vi "Autonomous Independent.vi"() -> ()   [LabVIEW 2016]
doc: "This VI is called when autonomous begins, and will automatically be terminated when autonomous ends. You can carry out timed or sensor driven robot movement independently without needing to return to the caller."
uses:
  <vilib>/Rock Robotics/WPI/Solenoid/WPI_SolenoidValue.ctl
  <vilib>/Rock Robotics/Network Tables/NT Read String.vi
  Robot Global Data.vi
  <vilib>/Rock Robotics/WPI/Solenoid/WPI_SolenoidSetEnum.vi
  <vilib>/Rock Robotics/WPI/Utilities/WPI_GetSetVariantRefNum.vi
  <vilib>/addons/control/pid/pid.llb/PID (DBL).vi
  <vilib>/addons/control/pid/NI_PID_pid.lvlib
  navX Library v2/navX Library v2.lvlib
panel:
  in  "ForwardPID":T1={"proportional gain (Kc)"=0.001, "integral time (Ti, min)"=0.1, "derivative time (Td, min)"=0.0}
  out "DriveStraight":T2(graph)
  in  "Center":dbl=180.0 format="%#_13g"
  in  "MOE":dbl=25.0 format="%#_13g"
  in  "Speed 2":dbl=0.45 format="%#_13g"
  in  "PID gains L":T1={"proportional gain (Kc)"=1.5e-05, "integral time (Ti, min)"=1e-07, "derivative time (Td, min)"=0.0} {"derivative time (Td, min)" format="%.3f"; "integral time (Ti, min)" format="%.6f"; "proportional gain (Kc)" format="%.6f"}
  in  "PID gains R":T1={"proportional gain (Kc)"=1.5e-05, "integral time (Ti, min)"=1e-07, "derivative time (Td, min)"=0.0} {"derivative time (Td, min)" format="%.3f"; "integral time (Ti, min)" format="%.6f"; "proportional gain (Kc)" format="%.6f"}
  in  "Range":cluster{"output high":dbl, "output low":dbl}={"output high"=1.0, "output low"=-1.0} {"output low" format="%.2f"; "output high" format="%.2f"}
  out "Right V":cluster{"output":dbl, dbl, "Numeric":dbl}(graph)
  out "Left V":cluster{"output":dbl, dbl, "Numeric":dbl}(graph)
  in  "Speed":dbl=1.0 format="%#_13g"
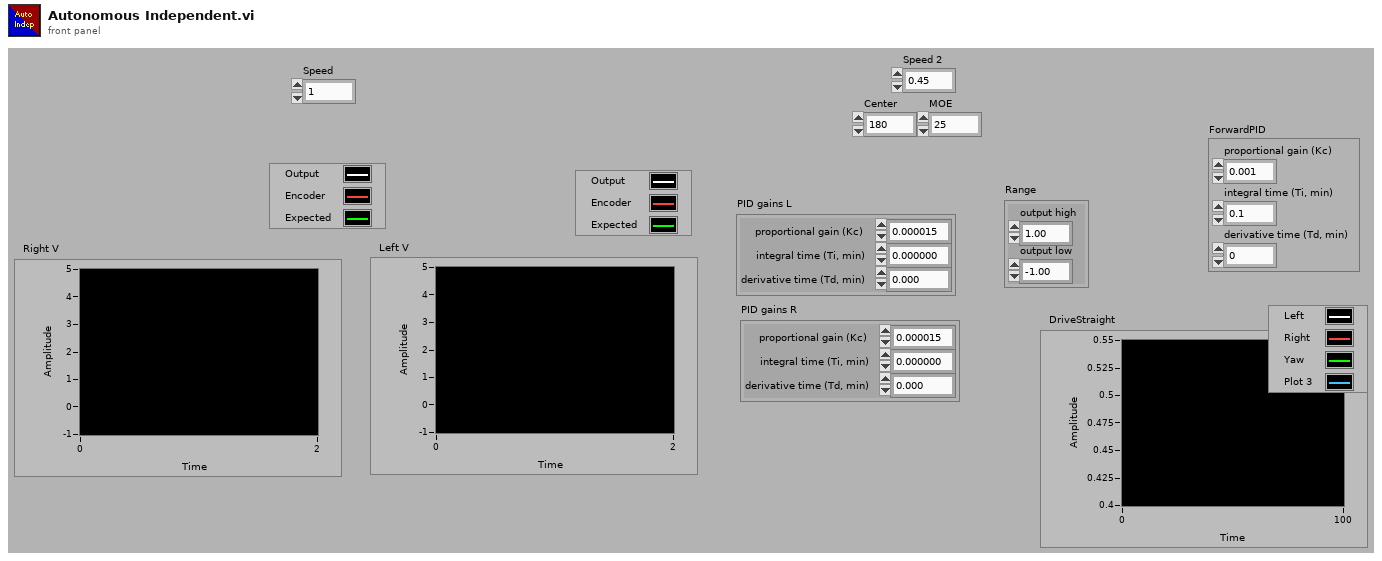
[diagram p1: front panel]
types:
  T1 = cluster{"proportional gain (Kc)":dbl, "integral time (Ti, min)":dbl, "derivative time (Td, min)":dbl}
  T2 = cluster{"[0]":dbl, "[1]":dbl, "[2]":dbl, "[3]":dbl, "[4]":dbl, "[5]":dbl, "[6]":dbl, "[7]":dbl, "[8]":dbl}
  T3 = typedef "WPI_SolenoidValue.ctl" = enum16{"Off", "On", "Forward", "Reverse"}
  T4 = typedef "WPI_SolenoidDevRef.ctl" = cluster{"DevStatus":errorcluster, "Pneumatics Control Module":u8, "Forward Solenoid Channel":T5, "Reverse Solenoid Channel":T5}
  T5 = typedef "WPI_SolenoidChannel.ctl" = enum8{"Solenoid 0", "Solenoid 1", "Solenoid 2", "Solenoid 3", "Solenoid 4", "Solenoid 5", "Solenoid 6", "Solenoid 7", "Invalid"}
  T6 = typedef "WPI_RobotDriveDevRef.ctl" = cluster{"DevStatus":errorcluster, "Motors[]":T7[], "Square Inputs":bool, "Max Output":dbl}
  T7 = typedef "WPI_MotorControlDeviceRef.ctl" = cluster{"DeviceStatus":errorcluster, "Type":T8, "PWM":cluster{"PWM Channel":T9, "DeadBand":T10}, "CAN":cluster{"Device Number":u8, "SetOutput VI Ref":variant, "GetOutput VI Ref":variant, "Enable VI Ref":variant, "Disable VI Ref":variant, "Data":variant}, "Invert":bool}
  T8 = typedef "WPI_MotorControlType.ctl" = enum16{"PWM", "CAN"}
  T9 = typedef "FPGA_DIOPWMChannel.ctl" = enum8{"PWM 0", "PWM 1", "PWM 2", "PWM 3", "PWM 4", "PWM 5", "PWM 6", "PWM 7", "PWM 8", "PWM 9", "PWM MXP 0", "PWM MXP 1", "PWM MXP 2", "PWM MXP 3", "PWM MXP 4", "PWM MXP 5", "PWM MXP 6", "PWM MXP 7", "PWM MXP 8", "PWM MXP 9", "Invalid"}
  T10 = typedef "WPI_PWMDeadband.ctl" = cluster{"Name":string, "maxPositivePwm":i32, "minPositivePwm":i32, "centerPwm":i32, "maxNegativePwm":i32, "minNegativePwm":i32, "angularRange":u16}
  T11 = typedef "navX Library v2.lvlib/Z900_navX_DeviceTypeDef.ctl" = cluster{"Interface":cluster{"Protocol":T12, "Update Rate (4Hz-100Hz)":u8, "navX Open TypeDef":variant}, "Notify Packet":refnum<notifier>, "Loop VI Refnum":refnum<vi>, "Ready to Close Occurrence Refnum":refnum<k4>}
  T12 = typedef "navX Library v2.lvlib/Z900_navX_ProtocolTypeDef.ctl" = enum16{"SERIAL", "I2C", "SPI"}
  T13 = typedef "WPI_EncoderDevRef.ctl" = cluster{"DevStatus":errorcluster, "EncoderIndex":T14, "CounterIndex":T15, "DistancePerCount":dbl, "Decoding Type":T16}
  T14 = typedef "FPGA_EncoderIdx.ctl" = enum8{"Enc 0", "Enc 1", "Enc 2", "Enc 3", "Enc 4", "Enc 5", "Enc 6", "Enc 7", "Invalid"}
  T15 = typedef "FPGA_CounterCtrSystemIndex.ctl" = enum8{"Ctr 0", "Ctr 1", "Ctr 2", "Ctr 3", "Ctr 4", "Ctr 5", "Ctr 6", "Ctr 7", "Invalid"}
  T16 = typedef "WPI_EncoderType.ctl" = enum16{"1x", "2x", "4x"}
  T17 = cluster{"Yaw":dbl, "Roll":dbl, "Pitch":dbl, "Heading":dbl, "Fused Heading":dbl}
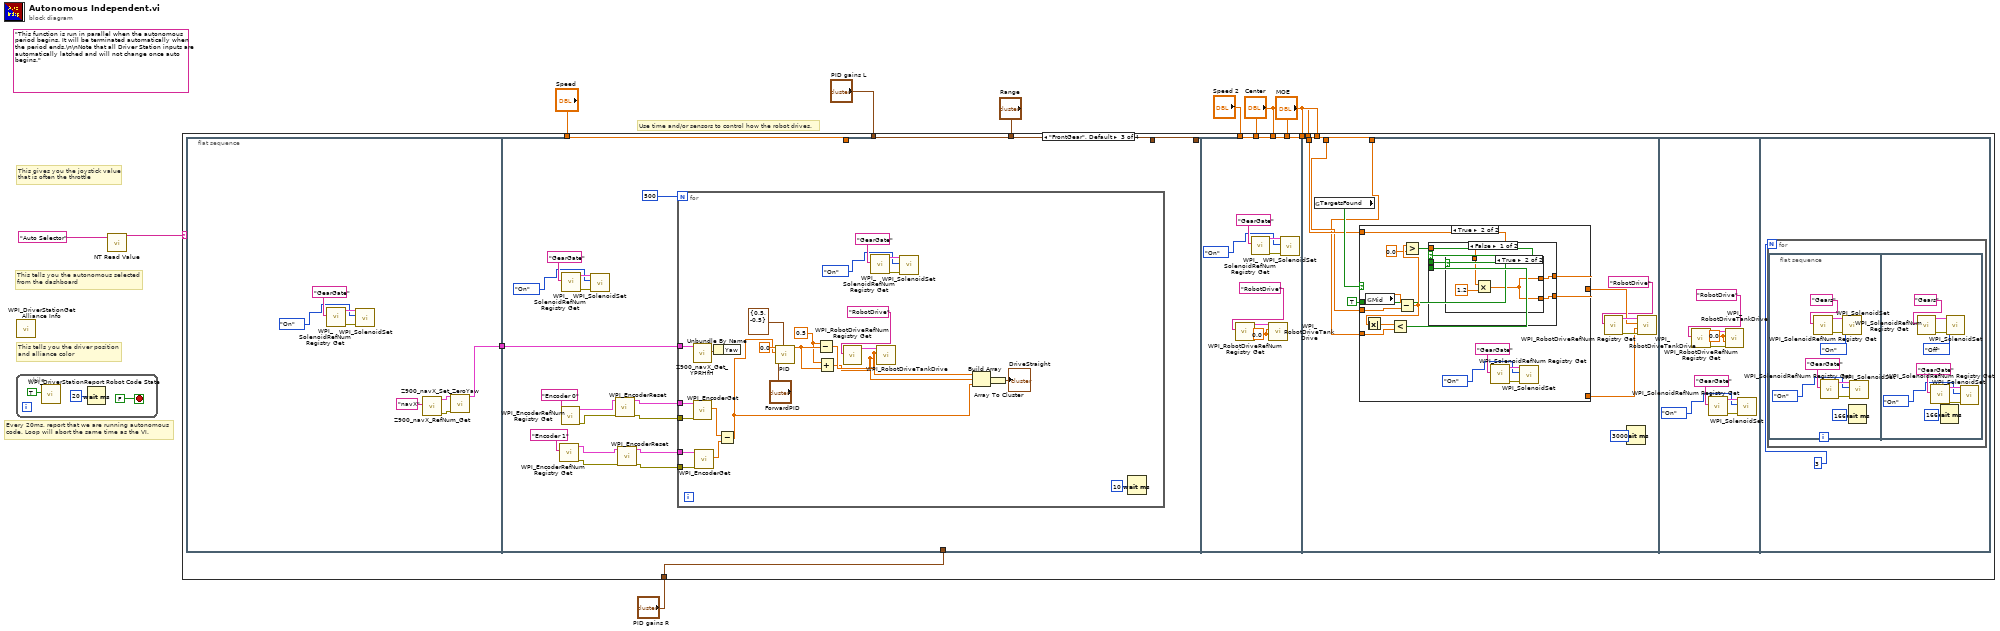
[diagram p0: block diagram]
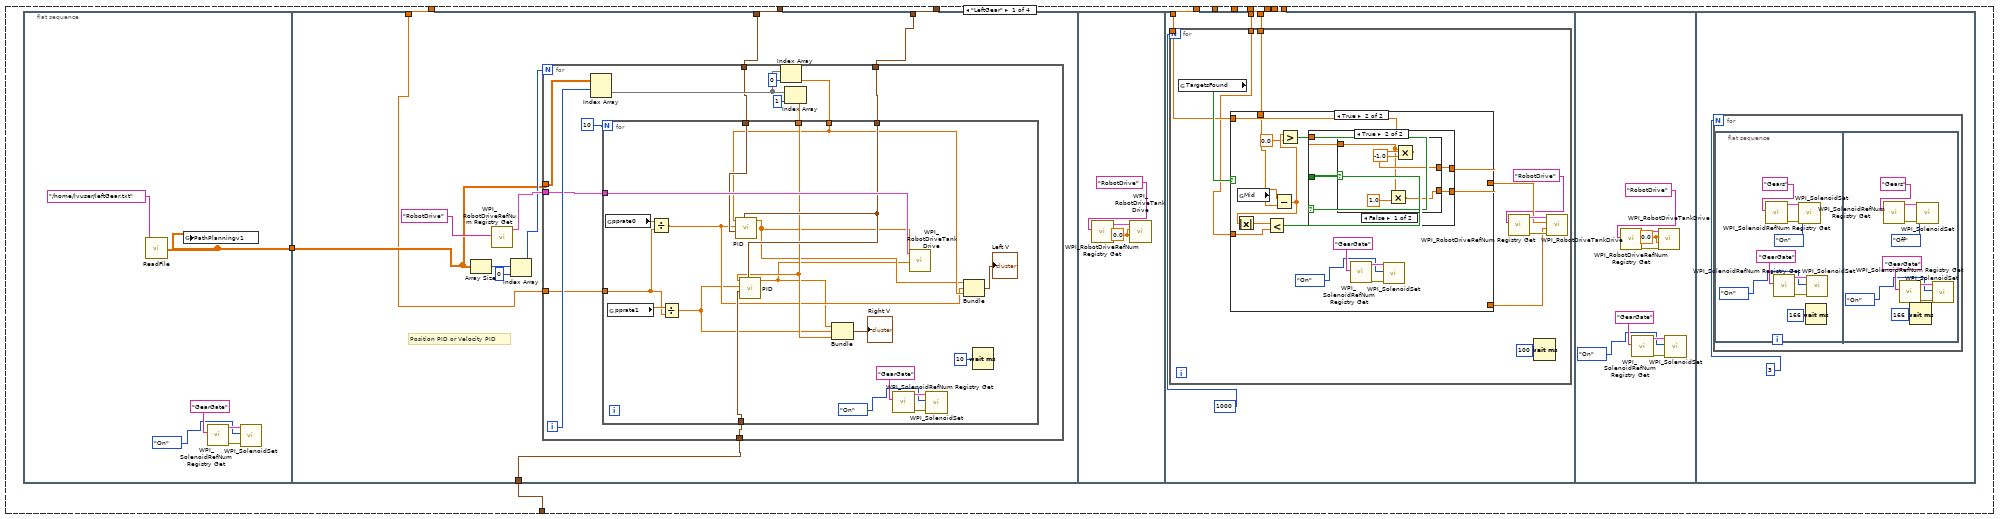
[diagram p2: hidden frame]
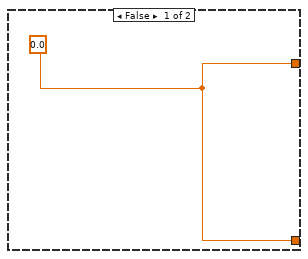
[diagram p3: hidden frame]
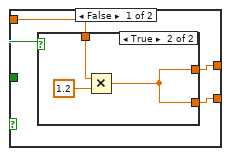
[diagram p4: hidden frame]
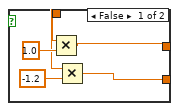
[diagram p5: hidden frame]
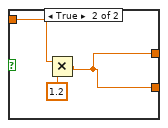
[diagram p6: hidden frame]
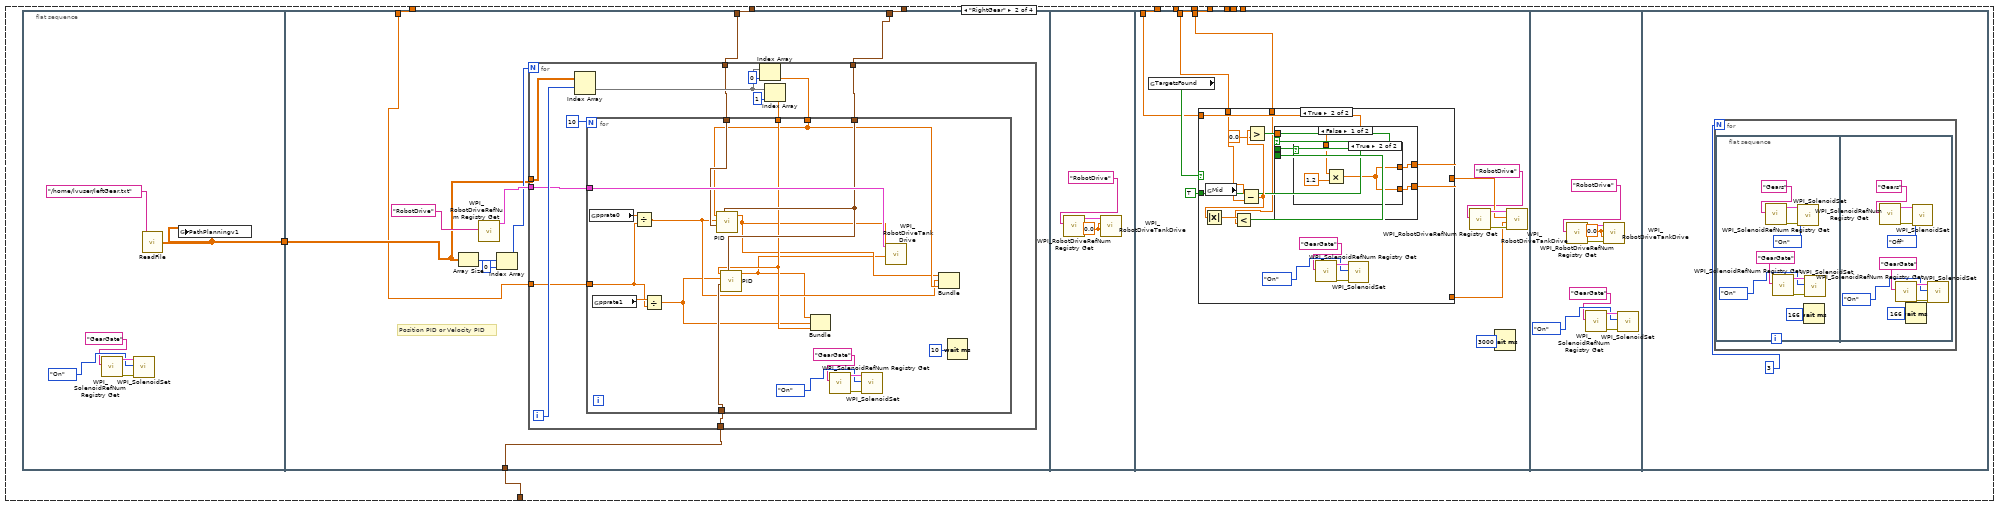
[diagram p7: hidden frame]
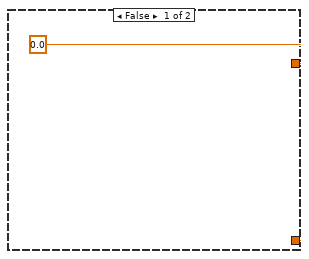
[diagram p8: hidden frame]
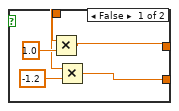
[diagram p9: hidden frame]
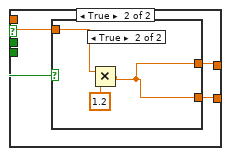
[diagram p10: hidden frame]
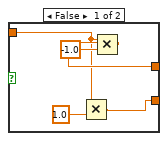
[diagram p11: hidden frame]
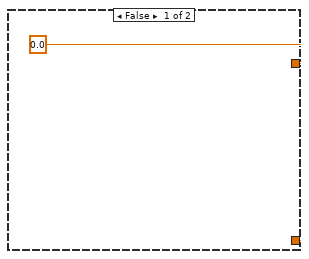
[diagram p12: hidden frame]
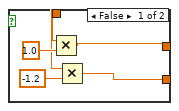
[diagram p13: hidden frame]
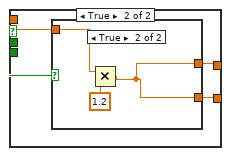
[diagram p14: hidden frame]
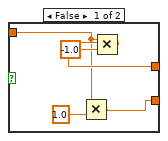
[diagram p15: hidden frame]
diagram:
  (unwired) "This function is run in parallel when the autonomous period begins. It will be terminated automatically when the period ends.\n\nNote that all Driver Station inputs are automatically latched and will not change once auto begins."
  # "This tells you the autonomous selected\nfrom the dashboard"
  # "Every 20ms, report that we are running autonomous\ncode. Loop will abort the same time as the VI."
  # "This gives you the joystick value\nthat is often the throttle"
  # "Use time and/or sensors to control how the robot drives."
  # "This tells you the driver position\nand alliance color"
  n1 = while {
    stop <- FALSE stop-if-true
    n2 = call <vilib>:"WPI_DriverStationReport Robot Code State.vi"("Autonomous"=TRUE) -> ()  [unwired: 10 in, 1 out]
    n3 = Wait (ms)(milliseconds to wait=u32 20) -> ()  [unwired: 1 out]
  }
  n4 = call <vilib>:"WPI_DriverStationGet Alliance Info.vi"() -> ()  [unwired: 12 out]
  n5 = call-poly <vilib>:"NT Read Value.vi"("Name"="Auto Selector") -> ("String"=w8:string)  [unwired: 9 in, 1 out]
  n6 = case shown="\"FrontGear\", Default" w8 {
    tunnel: "Range" -> [w19 w160 w298 _]
    tunnel: "PID gains L" -> [w18 w159 w297 _]
    tunnel: "Speed 2" -> [w17 w157 w296 _]
    tunnel: "Center" -> [w16 _ _ _]
    tunnel: "MOE" -> [w15 _ _ _]
    tunnel: "Speed" -> [w14 w158 w293 _]
    tunnel: "Center" -> [_ w156 _ _]
    tunnel: "MOE" -> [_ w155 _ _]
    tunnel: "Center" -> [_ _ w295 _]
    tunnel: "MOE" -> [_ _ w294 _]
    tunnel: "PID gains R" -> [w13 w154 w292 _]
    frame "LeftGear" {
      n7 = flat-sequence {
        tunnel: [w25] -> w20
        tunnel: w20 -> [w31]
        tunnel: w19 -> [w30]
        tunnel: w18 -> [w29]
        tunnel: w14 -> [w28]
        tunnel: w13 -> [w27]
        tunnel: w17 -> [w76]
        tunnel: w16 -> [w75]
        tunnel: w15 -> [w74]
        frame #0 {
          n8 = call "ReadFile.vi"("Name"="/home/lvuser/leftGear.txt") -> ("Array - Numeric"=w25:dbl[][])
          n9 = global write "Robot Global Data.vi" "PathPlanningv1"(w25) -> ()
          n10 = call <vilib>:"WPI_SolenoidRefNum Registry Get.vi"("refnum name"="GearGate") -> ("error out"=w24:errorcluster, "SolenoidDevRef"=w23:T4)  [unwired: 9 in]
          n11 = call-poly <vilib>:"WPI_SolenoidSet.vi"("error in (no error)"=w24, "Value"=WPI_SolenoidValue."On", "SolenoidDevRef"=w23) -> ()  [unwired: 7 in, 2 out]
        }
        frame #1 {
          # "Position PID or Velocity PID"
          n12 = Array Size(array=w31) -> (size(s)=w36:i32[])
          n13 = call <vilib>:"WPI_RobotDriveRefNum Registry Get.vi"("refnum name"="RobotDrive") -> ("RobotDriveDevRef"=w33:T6)  [unwired: 9 in, 1 out]
          n14 = Index Array(array=w36, index=0) -> (element=w32:i32)
          n15 = for {
            N: w32 -> [_]
            tunnel: w31 -> [w46]
            tunnel: w27 -> [w41]
            tunnel: w29 -> [w40]
            tunnel: w30 -> [w39]
            tunnel: w33 -> [w38]
            tunnel: w28 -> [w37]
            i -> [w43]
            n16 = Index Array(array=w46, index (row)=w43) -> (element=w49:dbl[])  [unwired: 1 in]
            n17 = Index Array(array=w49, index=0) -> (element=w45:dbl)
            n18 = Index Array(array=w49, index=1) -> (element=w44:dbl)
            n19 = for {
              N: 10 -> [_]
              tunnel: w45 -> [w63]
              tunnel: w44 -> [w64]
              tunnel: w41 -> [w67]
              tunnel: w40 -> [w66]
              tunnel: w39 -> [w65]
              tunnel: w38 -> [w68]
              tunnel: w37 -> [w56]
              n20 = global read "Robot Global Data.vi" "pprate0"() -> (w60:dbl)
              n21 = global read "Robot Global Data.vi" "pprate1"() -> (w57:dbl)
              n22 = Divide(x=w60, y=w56) -> (x/y=w59:dbl)
              n23 = Divide(x=w57, y=w56) -> (x/y=w58:dbl)
              n24 = call-poly <vilib>:"PID.vi"("output range"=w65, "PID gains"=w66, "process variable"=w59, "setpoint"=w63) -> ("output"=w55:dbl)  [unwired: 6 in, 1 out]
              n25 = call-poly <vilib>:"PID.vi"("output range"=w65, "PID gains"=w67, "process variable"=w58, "setpoint"=w64) -> ("output"=w54:dbl)  [unwired: 6 in, 1 out]
              n26 = Bundle("output"=w54, w58, "Numeric"=w64) -> (→"Right V":cluster{"output":dbl, dbl, "Numeric":dbl})  [unwired: 1 in]
              n27 = call <vilib>:"WPI_SolenoidRefNum Registry Get.vi"("refnum name"="GearGate") -> ("error out"=w53:errorcluster, "SolenoidDevRef"=w52:T4)  [unwired: 9 in]
              n28 = call <vilib>:"WPI_RobotDriveTankDrive.vi"("Right axis value"=w54, "Left axis value"=w55, "RobotDriveDevRef"=w68) -> ()  [unwired: 6 in, 3 out]
              n29 = call-poly <vilib>:"WPI_SolenoidSet.vi"("error in (no error)"=w53, "Value"=WPI_SolenoidValue."On", "SolenoidDevRef"=w52) -> ()  [unwired: 7 in, 2 out]
              n30 = Bundle("output"=w55, w59, "Numeric"=w63) -> (→"Left V":cluster{"output":dbl, dbl, "Numeric":dbl})  [unwired: 1 in]
              n31 = Wait (ms)(milliseconds to wait=10) -> ()  [unwired: 1 out]
            }
          }
        }
        frame #2 {
          w71 = 0.0 ("Right axis value")
          n32 = call <vilib>:"WPI_RobotDriveRefNum Registry Get.vi"("refnum name"="RobotDrive") -> ("RobotDriveDevRef"=w72:T6)  [unwired: 9 in, 1 out]
          n33 = call <vilib>:"WPI_RobotDriveTankDrive.vi"("Right axis value"=w71, "Left axis value"=w71, "RobotDriveDevRef"=w72) -> ()  [unwired: 6 in, 3 out]
        }
        frame #3 {
          n34 = for {
            N: 1000 -> [_]
            tunnel: w76 -> [w79]
            tunnel: w75 -> [w78]
            tunnel: w74 -> [w77]
            n35 = global read "Robot Global Data.vi" "TargetsFound"() -> (w80:bool)
            n36 = case shown="True" w80 {
              tunnel: [w87 w99] -> w83
              tunnel: [w87 w98] -> w84
              tunnel: w79 -> [_ w94]
              tunnel: w78 -> [_ w93]
              tunnel: w77 -> [_ w92]
              frame False {
                w87 = 0.0
              }
              frame True {
                n37 = global read "Robot Global Data.vi" "Mid"() -> (w102:dbl)
                n38 = Subtract(x=w102, y=w93) -> (x-y=w96:dbl)
                n39 = Absolute Value(x=w96) -> (abs(x)=w101:dbl)
                n40 = Less?(x=w101, y=w92) -> (x < y?=w100:bool)
                n41 = Greater?(x=w96, y=0.0) -> (0:w97:bool)
                n42 = case shown="True" w97 {
                  tunnel: w100 -> [w103 w118]
                  tunnel: [w104 w116] -> w99
                  tunnel: [w105 w117] -> w98
                  tunnel: w94 -> [w106 w115]
                  frame False {
                    n43 = case shown="True" w103 {
                      tunnel: [w111 w114] -> w105
                      tunnel: [w109 w114] -> w104
                      tunnel: w106 -> [w107 w112]
                      frame False {
                        n44 = Multiply(x=w107, y=1.0) -> (x*y=w111:dbl)
                        n45 = Multiply(x=w107, y=-1.2) -> (x*y=w109:dbl)
                      }
                      frame True {
                        n46 = Multiply(x=w112, y=1.2) -> (x*y=w114:dbl)
                      }
                    }
                  }
                  frame True {
                    n47 = case shown="False" w118 {
                      tunnel: [w123 w126] -> w117
                      tunnel: [w121 w126] -> w116
                      tunnel: w115 -> [w119 w124]
                      frame False {
                        n48 = Multiply(x=w119, y=1.0) -> (x*y=w121:dbl)
                        n49 = Multiply(x=w119, y=-1.0) -> (x*y=w123:dbl)
                      }
                      frame True {
                        n50 = Multiply(x=w124, y=1.2) -> (x*y=w126:dbl)
                      }
                    }
                  }
                }
                n51 = call <vilib>:"WPI_SolenoidRefNum Registry Get.vi"("refnum name"="GearGate") -> ("error out"=w91:errorcluster, "SolenoidDevRef"=w90:T4)  [unwired: 9 in]
                n52 = call-poly <vilib>:"WPI_SolenoidSet.vi"("error in (no error)"=w91, "Value"=WPI_SolenoidValue."On", "SolenoidDevRef"=w90) -> ()  [unwired: 7 in, 2 out]
              }
            }
            n53 = call <vilib>:"WPI_RobotDriveRefNum Registry Get.vi"("refnum name"="RobotDrive") -> ("error out"=w85:errorcluster, "RobotDriveDevRef"=w86:T6)  [unwired: 9 in]
            n54 = Wait (ms)(milliseconds to wait=100) -> ()  [unwired: 1 out]
            n55 = call <vilib>:"WPI_RobotDriveTankDrive.vi"("error in (no error)"=w85, "Right axis value"=w83, "Left axis value"=w84, "RobotDriveDevRef"=w86) -> ()  [unwired: 5 in, 3 out]
          }
        }
        frame #4 {
          w132 = 0.0 ("Left axis value")
          n56 = call <vilib>:"WPI_RobotDriveRefNum Registry Get.vi"("refnum name"="RobotDrive") -> ("error out"=w133:errorcluster, "RobotDriveDevRef"=w134:T6)  [unwired: 9 in]
          n57 = call <vilib>:"WPI_SolenoidRefNum Registry Get.vi"("refnum name"="GearGate") -> ("error out"=w130:errorcluster, "SolenoidDevRef"=w129:T4)  [unwired: 9 in]
          n58 = call <vilib>:"WPI_RobotDriveTankDrive.vi"("error in (no error)"=w133, "Right axis value"=w132, "Left axis value"=w132, "RobotDriveDevRef"=w134) -> ()  [unwired: 5 in, 3 out]
          n59 = call-poly <vilib>:"WPI_SolenoidSet.vi"("error in (no error)"=w130, "Value"=WPI_SolenoidValue."On", "SolenoidDevRef"=w129) -> ()  [unwired: 7 in, 2 out]
        }
        frame #5 {
          n60 = for {
            N: 3 -> [_]
            n61 = flat-sequence {
              frame #0 {
                n62 = call <vilib>:"WPI_SolenoidRefNum Registry Get.vi"("refnum name"="Gears") -> ("error out"=w144:errorcluster, "SolenoidDevRef"=w143:T4)  [unwired: 9 in]
                n63 = call <vilib>:"WPI_SolenoidRefNum Registry Get.vi"("refnum name"="GearGate") -> ("error out"=w139:errorcluster, "SolenoidDevRef"=w138:T4)  [unwired: 9 in]
                n64 = call-poly <vilib>:"WPI_SolenoidSet.vi"("error in (no error)"=w144, "Value"=WPI_SolenoidValue."On", "SolenoidDevRef"=w143) -> ()  [unwired: 7 in, 2 out]
                n65 = Wait (ms)(milliseconds to wait=166) -> ()  [unwired: 1 out]
                n66 = call-poly <vilib>:"WPI_SolenoidSet.vi"("error in (no error)"=w139, "Value"=WPI_SolenoidValue."On", "SolenoidDevRef"=w138) -> ()  [unwired: 7 in, 2 out]
              }
              frame #1 {
                n67 = call <vilib>:"WPI_SolenoidRefNum Registry Get.vi"("refnum name"="Gears") -> ("error out"=w153:errorcluster, "SolenoidDevRef"=w152:T4)  [unwired: 9 in]
                n68 = call <vilib>:"WPI_SolenoidRefNum Registry Get.vi"("refnum name"="GearGate") -> ("error out"=w148:errorcluster, "SolenoidDevRef"=w147:T4)  [unwired: 9 in]
                n69 = Wait (ms)(milliseconds to wait=166) -> ()  [unwired: 1 out]
                n70 = call-poly <vilib>:"WPI_SolenoidSet.vi"("error in (no error)"=w153, "Value"=WPI_SolenoidValue."Off", "SolenoidDevRef"=w152) -> ()  [unwired: 7 in, 2 out]
                n71 = call-poly <vilib>:"WPI_SolenoidSet.vi"("error in (no error)"=w148, "Value"=WPI_SolenoidValue."On", "SolenoidDevRef"=w147) -> ()  [unwired: 7 in, 2 out]
              }
            }
          }
        }
      }
    }
    frame "RightGear" {
      n72 = flat-sequence {
        tunnel: [w166] -> w161
        tunnel: w161 -> [w172]
        tunnel: w160 -> [w171]
        tunnel: w159 -> [w170]
        tunnel: w158 -> [w169]
        tunnel: w154 -> [w168]
        tunnel: w157 -> [w214]
        tunnel: w156 -> [w213]
        tunnel: w155 -> [w212]
        frame #0 {
          n73 = call <vilib>:"WPI_SolenoidRefNum Registry Get.vi"("refnum name"="GearGate") -> ("error out"=w165:errorcluster, "SolenoidDevRef"=w164:T4)  [unwired: 9 in]
          n74 = call-poly <vilib>:"WPI_SolenoidSet.vi"("error in (no error)"=w165, "Value"=WPI_SolenoidValue."On", "SolenoidDevRef"=w164) -> ()  [unwired: 7 in, 2 out]
          n75 = call "ReadFile.vi"("Name"="/home/lvuser/leftGear.txt") -> ("Array - Numeric"=w166:dbl[][])
          n76 = global write "Robot Global Data.vi" "PathPlanningv1"(w166) -> ()
        }
        frame #1 {
          # "Position PID or Velocity PID"
          n77 = Array Size(array=w172) -> (size(s)=w177:i32[])
          n78 = call <vilib>:"WPI_RobotDriveRefNum Registry Get.vi"("refnum name"="RobotDrive") -> ("RobotDriveDevRef"=w174:T6)  [unwired: 9 in, 1 out]
          n79 = Index Array(array=w177, index=0) -> (element=w173:i32)
          n80 = for {
            N: w173 -> [_]
            tunnel: w172 -> [w187]
            tunnel: w168 -> [w182]
            tunnel: w170 -> [w181]
            tunnel: w171 -> [w180]
            tunnel: w174 -> [w179]
            tunnel: w169 -> [w178]
            i -> [w184]
            n81 = Index Array(array=w187, index (row)=w184) -> (element=w190:dbl[])  [unwired: 1 in]
            n82 = Index Array(array=w190, index=0) -> (element=w186:dbl)
            n83 = Index Array(array=w190, index=1) -> (element=w185:dbl)
            n84 = for {
              N: 10 -> [_]
              tunnel: w186 -> [w202]
              tunnel: w185 -> [w203]
              tunnel: w182 -> [w206]
              tunnel: w181 -> [w205]
              tunnel: w180 -> [w204]
              tunnel: w179 -> [w207]
              tunnel: w178 -> [w197]
              n85 = global read "Robot Global Data.vi" "pprate0"() -> (w201:dbl)
              n86 = global read "Robot Global Data.vi" "pprate1"() -> (w198:dbl)
              n87 = Divide(x=w201, y=w197) -> (x/y=w200:dbl)
              n88 = Divide(x=w198, y=w197) -> (x/y=w199:dbl)
              n89 = call-poly <vilib>:"PID.vi"("output range"=w204, "PID gains"=w205, "process variable"=w200, "setpoint"=w202) -> ("output"=w196:dbl)  [unwired: 6 in, 1 out]
              n90 = call-poly <vilib>:"PID.vi"("output range"=w204, "PID gains"=w206, "process variable"=w199, "setpoint"=w203) -> ("output"=w195:dbl)  [unwired: 6 in, 1 out]
              n91 = Bundle("output"=w195, w199, "Numeric"=w203) -> ()  [unwired: 1 in, 1 out]
              n92 = call <vilib>:"WPI_SolenoidRefNum Registry Get.vi"("refnum name"="GearGate") -> ("error out"=w194:errorcluster, "SolenoidDevRef"=w193:T4)  [unwired: 9 in]
              n93 = call-poly <vilib>:"WPI_SolenoidSet.vi"("error in (no error)"=w194, "Value"=WPI_SolenoidValue."On", "SolenoidDevRef"=w193) -> ()  [unwired: 7 in, 2 out]
              n94 = call <vilib>:"WPI_RobotDriveTankDrive.vi"("Right axis value"=w195, "Left axis value"=w196, "RobotDriveDevRef"=w207) -> ()  [unwired: 6 in, 3 out]
              n95 = Bundle("output"=w196, w200, "Numeric"=w202) -> ()  [unwired: 1 in, 1 out]
              n96 = Wait (ms)(milliseconds to wait=10) -> ()  [unwired: 1 out]
            }
          }
        }
        frame #2 {
          w210 = 0.0 ("Right axis value")
          n97 = call <vilib>:"WPI_RobotDriveRefNum Registry Get.vi"("refnum name"="RobotDrive") -> ("RobotDriveDevRef"=w211:T6)  [unwired: 9 in, 1 out]
          n98 = call <vilib>:"WPI_RobotDriveTankDrive.vi"("Right axis value"=w210, "Left axis value"=w210, "RobotDriveDevRef"=w211) -> ()  [unwired: 6 in, 3 out]
        }
        frame #3 {
          n99 = global read "Robot Global Data.vi" "TargetsFound"() -> (w215:bool)
          n100 = case shown="True" w215 {
            tunnel: [w223 w236] -> w218
            tunnel: [w223 w235] -> w219
            tunnel: TRUE -> [_ w231]
            tunnel: w214 -> [_ w230]
            tunnel: w213 -> [_ w229]
            tunnel: w212 -> [_ w228]
            frame False {
              w223 = 0.0
            }
            frame True {
              n101 = global read "Robot Global Data.vi" "Mid"() -> (w239:dbl)
              n102 = Subtract(x=w239, y=w229) -> (x-y=w233:dbl)
              n103 = Absolute Value(x=w233) -> (abs(x)=w238:dbl)
              n104 = Less?(x=w238, y=w228) -> (x < y?=w237:bool)
              n105 = Greater?(x=w233, y=0.0) -> (0:w234:bool)
              n106 = case shown="False" w234 {
                tunnel: w237 -> [w240 w255]
                tunnel: [w241 w253] -> w236
                tunnel: [w242 w254] -> w235
                tunnel: w231 -> [_ _]
                tunnel: w230 -> [w243 w252]
                frame False {
                  n107 = case shown="True" w240 {
                    tunnel: [w248 w251] -> w242
                    tunnel: [w246 w251] -> w241
                    tunnel: w243 -> [w244 w249]
                    frame False {
                      n108 = Multiply(x=w244, y=1.0) -> (x*y=w248:dbl)
                      n109 = Multiply(x=w244, y=-1.2) -> (x*y=w246:dbl)
                    }
                    frame True {
                      n110 = Multiply(x=w249, y=1.2) -> (x*y=w251:dbl)
                    }
                  }
                }
                frame True {
                  n111 = case shown="True" w255 {
                    tunnel: [w260 w263] -> w254
                    tunnel: [w258 w263] -> w253
                    tunnel: w252 -> [w256 w261]
                    frame False {
                      n112 = Multiply(x=w256, y=1.0) -> (x*y=w258:dbl)
                      n113 = Multiply(x=w256, y=-1.0) -> (x*y=w260:dbl)
                    }
                    frame True {
                      n114 = Multiply(x=w261, y=1.2) -> (x*y=w263:dbl)
                    }
                  }
                }
              }
              n115 = call <vilib>:"WPI_SolenoidRefNum Registry Get.vi"("refnum name"="GearGate") -> ("error out"=w227:errorcluster, "SolenoidDevRef"=w226:T4)  [unwired: 9 in]
              n116 = call-poly <vilib>:"WPI_SolenoidSet.vi"("error in (no error)"=w227, "Value"=WPI_SolenoidValue."On", "SolenoidDevRef"=w226) -> ()  [unwired: 7 in, 2 out]
            }
          }
          n117 = call <vilib>:"WPI_RobotDriveRefNum Registry Get.vi"("refnum name"="RobotDrive") -> ("error out"=w220:errorcluster, "RobotDriveDevRef"=w221:T6)  [unwired: 9 in]
          n118 = Wait (ms)(milliseconds to wait=3000) -> ()  [unwired: 1 out]
          n119 = call <vilib>:"WPI_RobotDriveTankDrive.vi"("error in (no error)"=w220, "Right axis value"=w218, "Left axis value"=w219, "RobotDriveDevRef"=w221) -> ()  [unwired: 5 in, 3 out]
        }
        frame #4 {
          w269 = 0.0 ("Left axis value")
          n120 = call <vilib>:"WPI_RobotDriveRefNum Registry Get.vi"("refnum name"="RobotDrive") -> ("error out"=w270:errorcluster, "RobotDriveDevRef"=w271:T6)  [unwired: 9 in]
          n121 = call <vilib>:"WPI_SolenoidRefNum Registry Get.vi"("refnum name"="GearGate") -> ("error out"=w267:errorcluster, "SolenoidDevRef"=w266:T4)  [unwired: 9 in]
          n122 = call <vilib>:"WPI_RobotDriveTankDrive.vi"("error in (no error)"=w270, "Right axis value"=w269, "Left axis value"=w269, "RobotDriveDevRef"=w271) -> ()  [unwired: 5 in, 3 out]
          n123 = call-poly <vilib>:"WPI_SolenoidSet.vi"("error in (no error)"=w267, "Value"=WPI_SolenoidValue."On", "SolenoidDevRef"=w266) -> ()  [unwired: 7 in, 2 out]
        }
        frame #5 {
          n124 = for {
            N: 3 -> [_]
            n125 = flat-sequence {
              frame #0 {
                n126 = call <vilib>:"WPI_SolenoidRefNum Registry Get.vi"("refnum name"="Gears") -> ("error out"=w281:errorcluster, "SolenoidDevRef"=w280:T4)  [unwired: 9 in]
                n127 = call <vilib>:"WPI_SolenoidRefNum Registry Get.vi"("refnum name"="GearGate") -> ("error out"=w276:errorcluster, "SolenoidDevRef"=w275:T4)  [unwired: 9 in]
                n128 = call-poly <vilib>:"WPI_SolenoidSet.vi"("error in (no error)"=w281, "Value"=WPI_SolenoidValue."On", "SolenoidDevRef"=w280) -> ()  [unwired: 7 in, 2 out]
                n129 = Wait (ms)(milliseconds to wait=166) -> ()  [unwired: 1 out]
                n130 = call-poly <vilib>:"WPI_SolenoidSet.vi"("error in (no error)"=w276, "Value"=WPI_SolenoidValue."On", "SolenoidDevRef"=w275) -> ()  [unwired: 7 in, 2 out]
              }
              frame #1 {
                n131 = call <vilib>:"WPI_SolenoidRefNum Registry Get.vi"("refnum name"="Gears") -> ("error out"=w290:errorcluster, "SolenoidDevRef"=w289:T4)  [unwired: 9 in]
                n132 = call <vilib>:"WPI_SolenoidRefNum Registry Get.vi"("refnum name"="GearGate") -> ("error out"=w285:errorcluster, "SolenoidDevRef"=w284:T4)  [unwired: 9 in]
                n133 = Wait (ms)(milliseconds to wait=166) -> ()  [unwired: 1 out]
                n134 = call-poly <vilib>:"WPI_SolenoidSet.vi"("error in (no error)"=w290, "Value"=WPI_SolenoidValue."Off", "SolenoidDevRef"=w289) -> ()  [unwired: 7 in, 2 out]
                n135 = call-poly <vilib>:"WPI_SolenoidSet.vi"("error in (no error)"=w285, "Value"=WPI_SolenoidValue."On", "SolenoidDevRef"=w284) -> ()  [unwired: 7 in, 2 out]
              }
            }
          }
        }
      }
    }
    frame "FrontGear", Default {
      n136 = flat-sequence {
        tunnel: [w303] -> w291
        tunnel: w298 -> [_]
        tunnel: w297 -> [_]
        tunnel: w293 -> [_]
        tunnel: w292 -> [_]
        tunnel: w291 -> [w321]
        tunnel: w296 -> [w357]
        tunnel: w295 -> [w356]
        tunnel: w294 -> [w355]
        frame #0 {
          n137 = call <vilib>:"WPI_SolenoidRefNum Registry Get.vi"("refnum name"="GearGate") -> ("error out"=w302:errorcluster, "SolenoidDevRef"=w301:T4)  [unwired: 9 in]
          n138 = call-poly <vilib>:"WPI_SolenoidSet.vi"("error in (no error)"=w302, "Value"=WPI_SolenoidValue."On", "SolenoidDevRef"=w301) -> ()  [unwired: 7 in, 2 out]
          n139 = call "Z900_navX_RefNum_Get.vi"("refnum name"="navX") -> ("error out"=w305:errorcluster, "navX Device"=w306:T11)  [unwired: 9 in]
          n140 = call "Z900_navX_Set_ZeroYaw.vi"("error in (no error)"=w305, "navX Device"=w306) -> ("navX Device"=w303:T11)  [unwired: 8 in, 1 out]
        }
        frame #1 {
          n141 = call <vilib>:"WPI_EncoderRefNum Registry Get.vi"("refnum name"="Encoder 1") -> ("error out"=w312:errorcluster, "EncoderDevRef"=w316:T13)  [unwired: 9 in]
          n142 = call <vilib>:"WPI_EncoderRefNum Registry Get.vi"("refnum name"="Encoder 0") -> ("error out"=w314:errorcluster, "EncoderDevRef"=w318:T13)  [unwired: 9 in]
          n143 = call <vilib>:"WPI_SolenoidRefNum Registry Get.vi"("refnum name"="GearGate") -> ("error out"=w310:errorcluster, "SolenoidDevRef"=w309:T4)  [unwired: 9 in]
          n144 = call-poly <vilib>:"WPI_SolenoidSet.vi"("error in (no error)"=w310, "Value"=WPI_SolenoidValue."On", "SolenoidDevRef"=w309) -> ()  [unwired: 7 in, 2 out]
          n145 = call <vilib>:"WPI_EncoderReset.vi"("error in (no error)"=w314, "EncoderDevRef"=w318) -> ("error out"=w313:errorcluster, "EncoderDevRef"=w317:T13)  [unwired: 8 in]
          n146 = call <vilib>:"WPI_EncoderReset.vi"("error in (no error)"=w312, "EncoderDevRef"=w316) -> ("error out"=w311:errorcluster, "EncoderDevRef"=w315:T13)  [unwired: 8 in]
          n147 = for {
            N: 500 -> [_]
            tunnel: w321 -> [w342]
            tunnel: w317 -> [w335]
            tunnel: w315 -> [w334]
            tunnel: w313 -> [w328]
            tunnel: w311 -> [w327]
            w344 = 0.5
            n148 = call "Z900_navX_Get_YPRHfH.vi"("navX Device"=w342) -> ("YRPHfH"=w341:T17)  [unwired: 7 in, 3 out]
            n149 = call <vilib>:"WPI_EncoderGet.vi"("error in (no error)"=w328, "EncoderDevRef"=w335) -> ("Distance"=w333:dbl)  [unwired: 4 in, 5 out]
            n150 = call <vilib>:"WPI_EncoderGet.vi"("error in (no error)"=w327, "EncoderDevRef"=w334) -> ("Distance"=w332:dbl)  [unwired: 4 in, 5 out]
            n151 = Unbundle By Name(w341) -> ()  [unwired: 1 out]
            n152 = Subtract(x=w333, y=w332) -> (x-y=w331:dbl)
            n153 = call-poly <vilib>:"PID.vi"("output range"=cluster{"output high":dbl, "output low":dbl} {"output high"=0.5, "output low"=-0.5}, "PID gains"="ForwardPID", "process variable"=w331, "setpoint"=0.0) -> ("output"=w345:dbl)  [unwired: 6 in, 1 out]
            n154 = Subtract(x=w344, y=w345) -> (x-y=w337:dbl)
            n155 = Add(x=w344, y=w345) -> (x+y=w336:dbl)
            n156 = call <vilib>:"WPI_RobotDriveRefNum Registry Get.vi"("refnum name"="RobotDrive") -> ("RobotDriveDevRef"=w347:T6)  [unwired: 9 in, 1 out]
            n157 = call <vilib>:"WPI_SolenoidRefNum Registry Get.vi"("refnum name"="GearGate") -> ("error out"=w326:errorcluster, "SolenoidDevRef"=w325:T4)  [unwired: 9 in]
            n158 = call <vilib>:"WPI_RobotDriveTankDrive.vi"("Right axis value"=w336, "Left axis value"=w337, "RobotDriveDevRef"=w347) -> ()  [unwired: 6 in, 3 out]
            n159 = call-poly <vilib>:"WPI_SolenoidSet.vi"("error in (no error)"=w326, "Value"=WPI_SolenoidValue."On", "SolenoidDevRef"=w325) -> ()  [unwired: 7 in, 2 out]
            n160 = Build Array(w337, w336, w331) -> (w329:dbl[])
            n161 = Array To Cluster(array=w329) -> (cluster=→"DriveStraight":T2)
            n162 = Wait (ms)(milliseconds to wait=10) -> ()  [unwired: 1 out]
          }
        }
        frame #2 {
          w353 = 0.0 ("Right axis value")
          n163 = call <vilib>:"WPI_RobotDriveRefNum Registry Get.vi"("refnum name"="RobotDrive") -> ("RobotDriveDevRef"=w354:T6)  [unwired: 9 in, 1 out]
          n164 = call <vilib>:"WPI_SolenoidRefNum Registry Get.vi"("refnum name"="GearGate") -> ("error out"=w351:errorcluster, "SolenoidDevRef"=w350:T4)  [unwired: 9 in]
          n165 = call <vilib>:"WPI_RobotDriveTankDrive.vi"("Right axis value"=w353, "Left axis value"=w353, "RobotDriveDevRef"=w354) -> ()  [unwired: 6 in, 3 out]
          n166 = call-poly <vilib>:"WPI_SolenoidSet.vi"("error in (no error)"=w351, "Value"=WPI_SolenoidValue."On", "SolenoidDevRef"=w350) -> ()  [unwired: 7 in, 2 out]
        }
        frame #3 {
          n167 = global read "Robot Global Data.vi" "TargetsFound"() -> (w358:bool)
          n168 = case shown="True" w358 {
            tunnel: [w366 w379] -> w361
            tunnel: [w366 w378] -> w362
            tunnel: TRUE -> [_ w374]
            tunnel: w357 -> [_ w373]
            tunnel: w356 -> [_ w372]
            tunnel: w355 -> [_ w371]
            frame False {
              w366 = 0.0
            }
            frame True {
              n169 = global read "Robot Global Data.vi" "Mid"() -> (w382:dbl)
              n170 = Subtract(x=w382, y=w372) -> (x-y=w376:dbl)
              n171 = Absolute Value(x=w376) -> (abs(x)=w381:dbl)
              n172 = Less?(x=w381, y=w371) -> (x < y?=w380:bool)
              n173 = Greater?(x=w376, y=0.0) -> (0:w377:bool)
              n174 = case shown="False" w377 {
                tunnel: w380 -> [w383 w398]
                tunnel: [w384 w396] -> w379
                tunnel: [w385 w397] -> w378
                tunnel: w374 -> [_ _]
                tunnel: w373 -> [w386 w395]
                frame False {
                  n175 = case shown="True" w383 {
                    tunnel: [w391 w394] -> w385
                    tunnel: [w389 w394] -> w384
                    tunnel: w386 -> [w387 w392]
                    frame False {
                      n176 = Multiply(x=w387, y=1.0) -> (x*y=w391:dbl)
                      n177 = Multiply(x=w387, y=-1.2) -> (x*y=w389:dbl)
                    }
                    frame True {
                      n178 = Multiply(x=w392, y=1.2) -> (x*y=w394:dbl)
                    }
                  }
                }
                frame True {
                  n179 = case shown="True" w398 {
                    tunnel: [w403 w406] -> w397
                    tunnel: [w401 w406] -> w396
                    tunnel: w395 -> [w399 w404]
                    frame False {
                      n180 = Multiply(x=w399, y=1.0) -> (x*y=w401:dbl)
                      n181 = Multiply(x=w399, y=-1.0) -> (x*y=w403:dbl)
                    }
                    frame True {
                      n182 = Multiply(x=w404, y=1.2) -> (x*y=w406:dbl)
                    }
                  }
                }
              }
              n183 = call <vilib>:"WPI_SolenoidRefNum Registry Get.vi"("refnum name"="GearGate") -> ("error out"=w370:errorcluster, "SolenoidDevRef"=w369:T4)  [unwired: 9 in]
              n184 = call-poly <vilib>:"WPI_SolenoidSet.vi"("error in (no error)"=w370, "Value"=WPI_SolenoidValue."On", "SolenoidDevRef"=w369) -> ()  [unwired: 7 in, 2 out]
            }
          }
          n185 = call <vilib>:"WPI_RobotDriveRefNum Registry Get.vi"("refnum name"="RobotDrive") -> ("error out"=w363:errorcluster, "RobotDriveDevRef"=w364:T6)  [unwired: 9 in]
          n186 = Wait (ms)(milliseconds to wait=3000) -> ()  [unwired: 1 out]
          n187 = call <vilib>:"WPI_RobotDriveTankDrive.vi"("error in (no error)"=w363, "Right axis value"=w361, "Left axis value"=w362, "RobotDriveDevRef"=w364) -> ()  [unwired: 5 in, 3 out]
        }
        frame #4 {
          w412 = 0.0 ("Left axis value")
          n188 = call <vilib>:"WPI_RobotDriveRefNum Registry Get.vi"("refnum name"="RobotDrive") -> ("error out"=w413:errorcluster, "RobotDriveDevRef"=w414:T6)  [unwired: 9 in]
          n189 = call <vilib>:"WPI_SolenoidRefNum Registry Get.vi"("refnum name"="GearGate") -> ("error out"=w410:errorcluster, "SolenoidDevRef"=w409:T4)  [unwired: 9 in]
          n190 = call <vilib>:"WPI_RobotDriveTankDrive.vi"("error in (no error)"=w413, "Right axis value"=w412, "Left axis value"=w412, "RobotDriveDevRef"=w414) -> ()  [unwired: 5 in, 3 out]
          n191 = call-poly <vilib>:"WPI_SolenoidSet.vi"("error in (no error)"=w410, "Value"=WPI_SolenoidValue."On", "SolenoidDevRef"=w409) -> ()  [unwired: 7 in, 2 out]
        }
        frame #5 {
          n192 = for {
            N: 3 -> [_]
            n193 = flat-sequence {
              frame #0 {
                n194 = call <vilib>:"WPI_SolenoidRefNum Registry Get.vi"("refnum name"="Gears") -> ("error out"=w424:errorcluster, "SolenoidDevRef"=w423:T4)  [unwired: 9 in]
                n195 = call <vilib>:"WPI_SolenoidRefNum Registry Get.vi"("refnum name"="GearGate") -> ("error out"=w419:errorcluster, "SolenoidDevRef"=w418:T4)  [unwired: 9 in]
                n196 = call-poly <vilib>:"WPI_SolenoidSet.vi"("error in (no error)"=w424, "Value"=WPI_SolenoidValue."On", "SolenoidDevRef"=w423) -> ()  [unwired: 7 in, 2 out]
                n197 = Wait (ms)(milliseconds to wait=166) -> ()  [unwired: 1 out]
                n198 = call-poly <vilib>:"WPI_SolenoidSet.vi"("error in (no error)"=w419, "Value"=WPI_SolenoidValue."On", "SolenoidDevRef"=w418) -> ()  [unwired: 7 in, 2 out]
              }
              frame #1 {
                n199 = call <vilib>:"WPI_SolenoidRefNum Registry Get.vi"("refnum name"="Gears") -> ("error out"=w433:errorcluster, "SolenoidDevRef"=w432:T4)  [unwired: 9 in]
                n200 = call <vilib>:"WPI_SolenoidRefNum Registry Get.vi"("refnum name"="GearGate") -> ("error out"=w428:errorcluster, "SolenoidDevRef"=w427:T4)  [unwired: 9 in]
                n201 = Wait (ms)(milliseconds to wait=166) -> ()  [unwired: 1 out]
                n202 = call-poly <vilib>:"WPI_SolenoidSet.vi"("error in (no error)"=w433, "Value"=WPI_SolenoidValue."Off", "SolenoidDevRef"=w432) -> ()  [unwired: 7 in, 2 out]
                n203 = call-poly <vilib>:"WPI_SolenoidSet.vi"("error in (no error)"=w428, "Value"=WPI_SolenoidValue."On", "SolenoidDevRef"=w427) -> ()  [unwired: 7 in, 2 out]
              }
            }
          }
        }
      }
    }
    frame "Nothing" {
    }
  }
